vi "TestExec.Config, Read Test Data Dir Info.vi"(8 "error in":errorcluster, 9 "Dirs In":T1[](array[typedef]), 11 "Station Data Dir Config File":path) -> (0 "error out":errorcluster, 1 "Working Dirs":T1[](array[typedef]), 2 "ResultExt":path, 3 "ResultLocal":path, 4 "Seq Result Dirs":T1[](array[typedef]))   [LabVIEW 2018]
uses:
  Common/Utils/TestExec/TestExec.WorkingDir.ctl
  <vilib>/Utility/config.llb/Read Key (String).vi
  <vilib>/Utility/config.llb/NI_LVConfig.lvlib
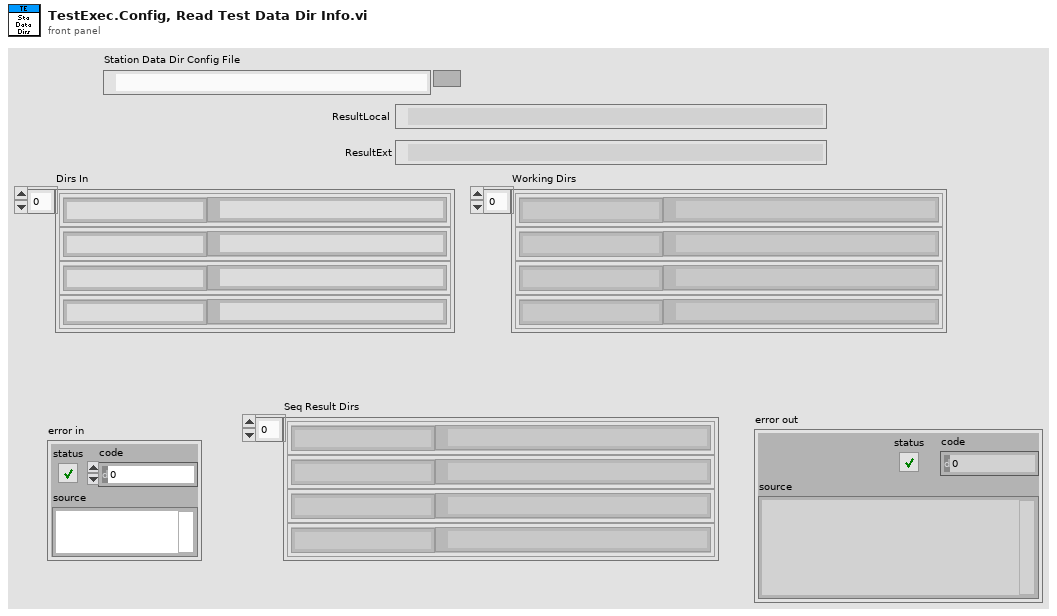
[diagram p1: front panel]
types:
  T1 = typedef "TestExec.WorkingDir.ctl" = cluster{"Name":string, "Path":path}
  T2 = typedef "NI_LVConfig.lvlib/Config Data RefNum.ctl" = refnum<k1>
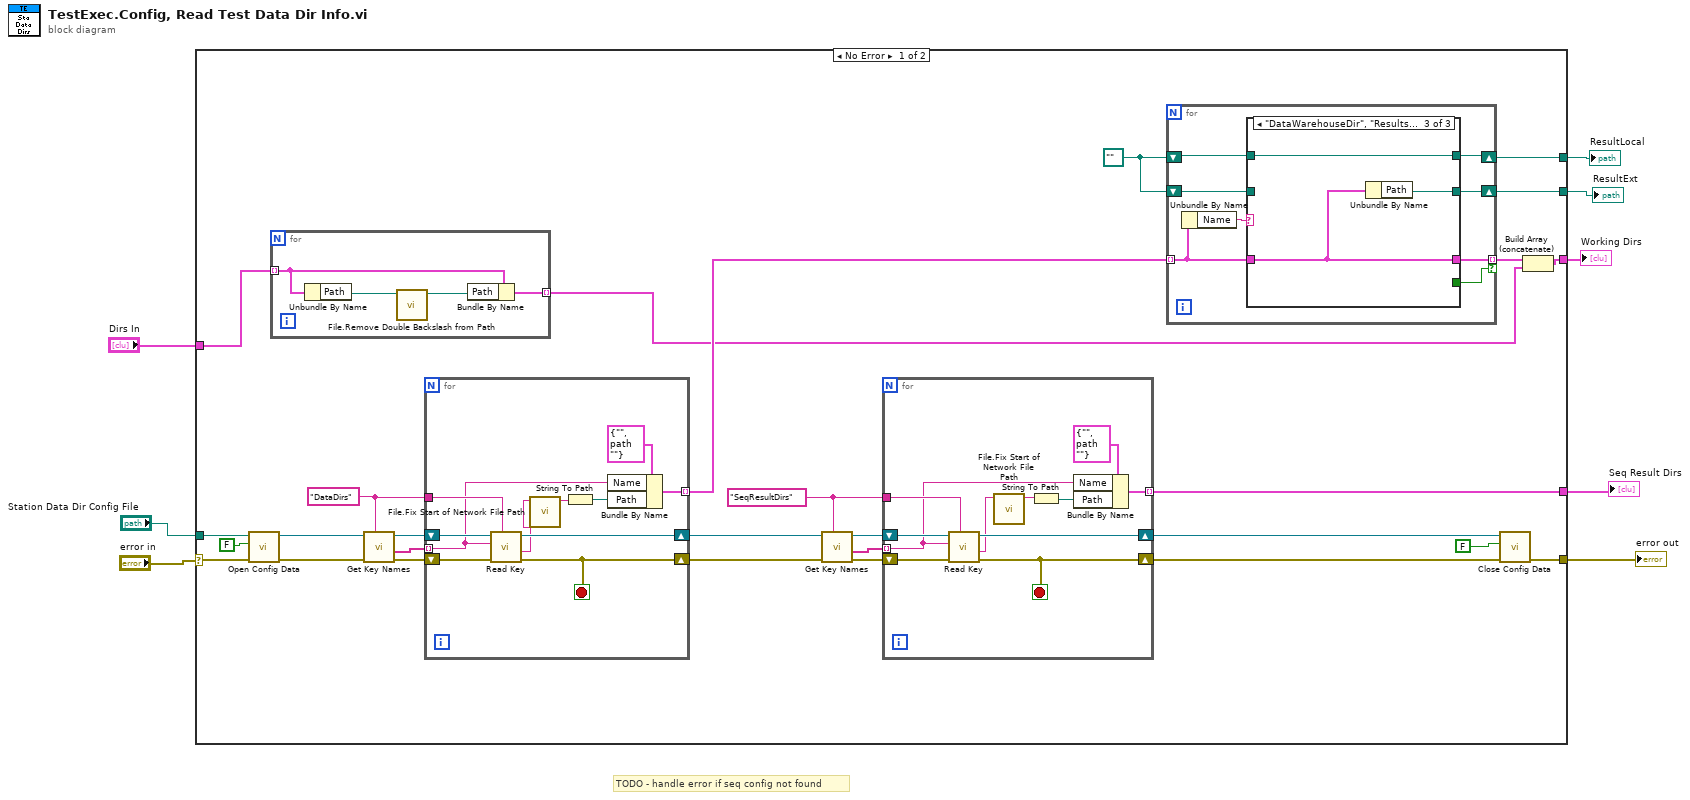
[diagram p0: block diagram]
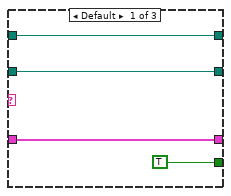
[diagram p2: hidden frame]
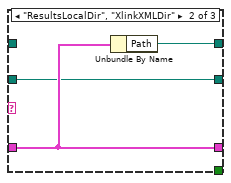
[diagram p3: hidden frame]
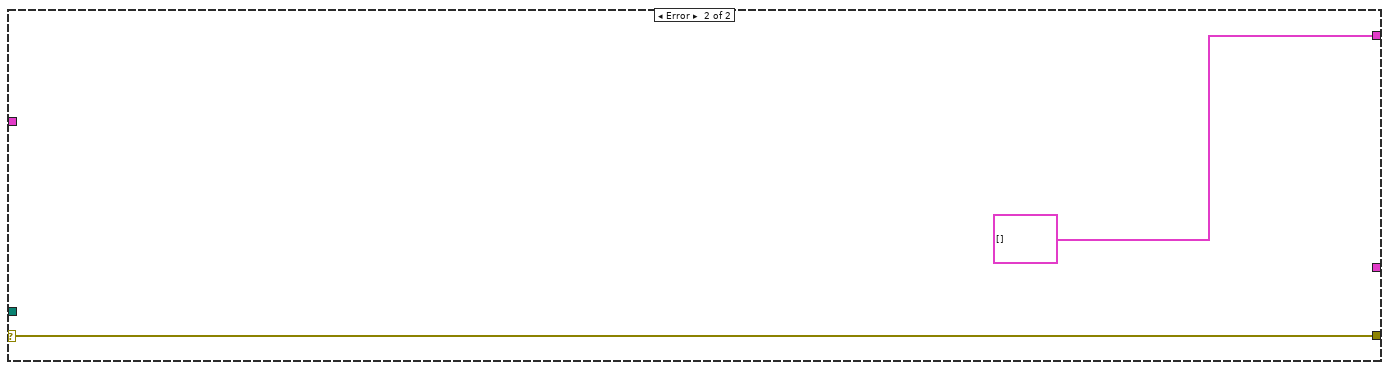
[diagram p4: hidden frame]
diagram:
  # "TODO - handle error if seq config not found"
  n1 = case shown="No Error" "error in" {
    selector: "error in" -> [w32 w82]
    tunnel: "Station Data Dir Config File" -> [w36 _]
    tunnel: [w35 w82] -> w7
    tunnel: [w21 T1[] []] -> w3
    tunnel: [w24 _] -> w4
    tunnel: [w23 _] -> w5
    tunnel: "Dirs In" -> [w10 _]
    tunnel: [w11 _] -> w1
    frame No Error {
      w19 = "SeqResultDirs"
      w25 = path ""
      w26 = "DataDirs"
      n2 = call <vilib>:"Open Config Data.vi"("error in (no error)"=w32, "create file if necessary (T)"=FALSE, "configuration file path"=w36) -> ("error out"=w30:errorcluster, "refnum"=w31:T2)  [unwired: 6 in, 1 out]
      n3 = for {
        tunnel: w10 -> [w40] mode=indexing
        tunnel: [w37] -> w9 mode=indexing
        n4 = Unbundle By Name(w40) -> ("Path"=w39:path)
        n5 = call "File.Remove Double Backslash from Path.vi"("Path"=w39) -> ("Path Out"=w38:path)  [unwired: 10 in]
        n6 = Bundle By Name(cluster=w40, "Path"=w38) -> (w37:T1)
      }
      n7 = call <vilib>:"Get Key Names.vi"("section"=w26, "error in (no error)"=w30, "refnum"=w31) -> ("error out"=w28:errorcluster, "key names"=w27:string[], "refnum out"=w29:T2)  [unwired: 5 in, 1 out]
      n8 = for {
        tunnel: w27 -> [w76] mode=indexing
        tunnel: w26 -> [w78]
        tunnel: [w75] -> w20 mode=indexing
        shift-right: [w73] -> w15
        shift-left: w29 -> [w80]
        shift-right: [w74] -> w14
        shift-left: w28 -> [w79]
        stop <- w74 stop-if-true
        n9 = call-poly <vilib>:"Read Key.vi"("section"=w78, "error in (no error)"=w79, "key"=w76, "refnum"=w80) -> ("error out"=w74:errorcluster, "value"=w70:string, "refnum out"=w73:T2)  [unwired: 4 in, 1 out]
        n10 = call "File.Fix Start of Network File Path.vi"("String Path"=w70) -> ("String Path Out"=w71:string)  [unwired: 10 in]
        n11 = String To Path(string=w71) -> (path=w72:path)
        n12 = Bundle By Name(cluster=T1 {"Name"="", "Path"=path ""} ("Working Dirs"), "Name"=w76, "Path"=w72) -> (w75:T1)
      }
      n13 = call <vilib>:"Get Key Names.vi"("section"=w19, "error in (no error)"=w14, "refnum"=w15) -> ("error out"=w17:errorcluster, "key names"=w18:string[], "refnum out"=w16:T2)  [unwired: 5 in, 1 out]
      n14 = for {
        tunnel: w18 -> [w47] mode=indexing
        tunnel: w19 -> [w49]
        tunnel: [w46] -> w11 mode=indexing
        shift-right: [w44] -> w12
        shift-left: w16 -> [w51]
        shift-right: [w45] -> w13
        shift-left: w17 -> [w50]
        stop <- w45 stop-if-true
        n15 = call-poly <vilib>:"Read Key.vi"("section"=w49, "error in (no error)"=w50, "key"=w47, "refnum"=w51) -> ("error out"=w45:errorcluster, "value"=w41:string, "refnum out"=w44:T2)  [unwired: 4 in, 1 out]
        n16 = call "File.Fix Start of Network File Path.vi"("String Path"=w41) -> ("String Path Out"=w42:string)  [unwired: 10 in]
        n17 = String To Path(string=w42) -> (path=w43:path)
        n18 = Bundle By Name(cluster=T1 {"Name"="", "Path"=path ""} ("Working Dirs"), "Name"=w47, "Path"=w43) -> (w46:T1)
      }
      n19 = for {
        tunnel: w20 -> [w59] mode=indexing
        shift-right: [w56] -> w23
        shift-left: w25 -> [w53]
        shift-right: [w54] -> w24
        shift-left: w25 -> [w55]
        tunnel: [w58] -> w22 mode=indexing if=w52
        n20 = Unbundle By Name(w59) -> ("Name"=w57:string)
        n21 = case shown="\"DataWarehouseDir\", \"ResultsExternalDir\"" w57 {
          tunnel: w59 -> [w63 w66 w69]
          tunnel: [w63 w66 w69] -> w58
          tunnel: [w62 w65 w67] -> w56
          tunnel: w55 -> [w61 w64 _]
          tunnel: [w61 w64 w68] -> w54
          tunnel: w53 -> [w62 _ w67]
          tunnel: [TRUE _ _] -> w52
          frame Default {
          }
          frame "ResultsLocalDir", "XlinkXMLDir" {
            n22 = Unbundle By Name(w66) -> ("Path"=w65:path)
          }
          frame "DataWarehouseDir", "ResultsExternalDir" {
            n23 = Unbundle By Name(w69) -> ("Path"=w68:path)
          }
        }
      }
      n24 = call <vilib>:"Close Config Data.vi"("error in (no error)"=w13, "write file if changed (T)"=FALSE, "refnum"=w12) -> ("error out"=w35:errorcluster)  [unwired: 7 in, 1 out]
      n25 = Build Array (concatenate)(w22, w9) -> (w21:T1[])
    }
    frame Error {
    }
  }
  "error out" <- w7
  "ResultLocal" <- w5
  "ResultExt" <- w4
  "Working Dirs" <- w3
  "Seq Result Dirs" <- w1
